vi "LoadIRF.vi"(8 "error in (no error)":errorcluster, 11 "file path":path=path "C:/Users/MarcuAdmin/Documents/GitHub/NetDeconForLV/Testing/irf files/Channel1.tdms") -> (0 "error out":errorcluster, 3 "APD":T1)   [LabVIEW 2020]
uses:
  APD.ctl
  <vilib>/Utility/TDMS File Viewer/NI_TDMS File Viewer.lvlib
panel:
  out "WFLength":i32
  out "Waveform Graph":dbl[][](graph)
  out "XY Graph":cluster{dbl[], dbl[]}(graph)
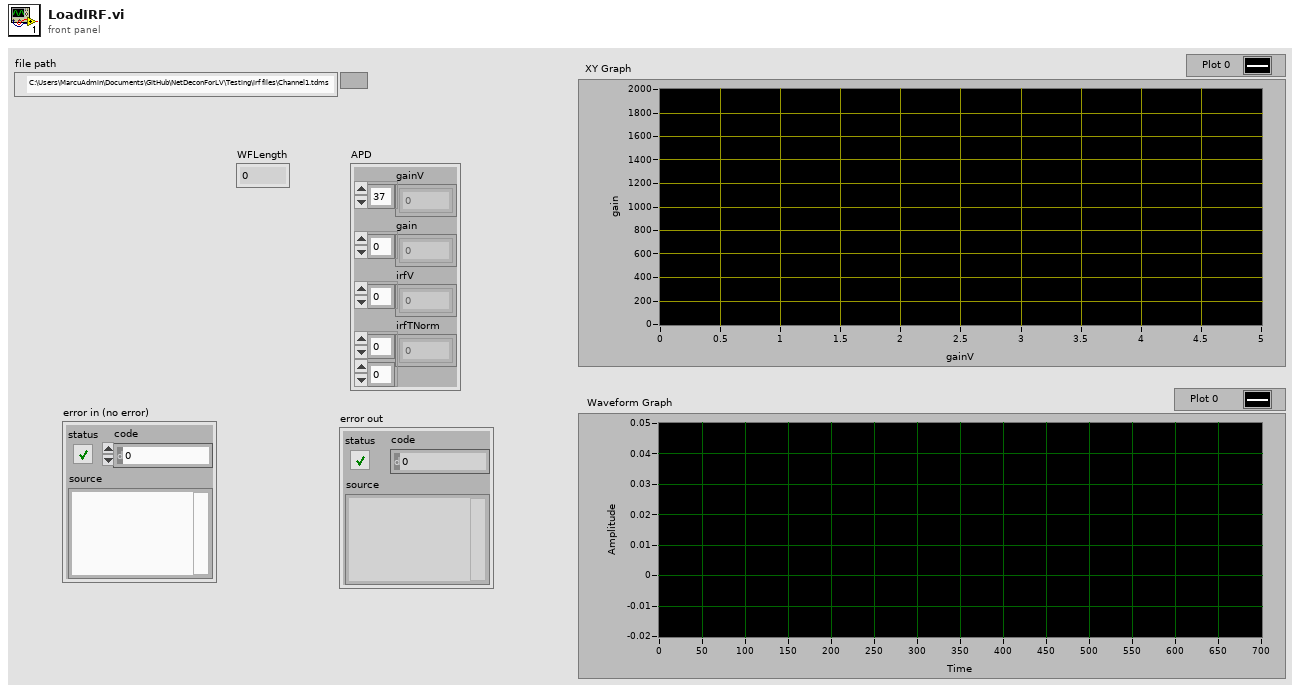
[diagram p1: front panel]
types:
  T1 = typedef "APD.ctl" = cluster{"gainV":dbl[], "gain":dbl[], "irfV":dbl[], "irfTNorm":dbl[][]}
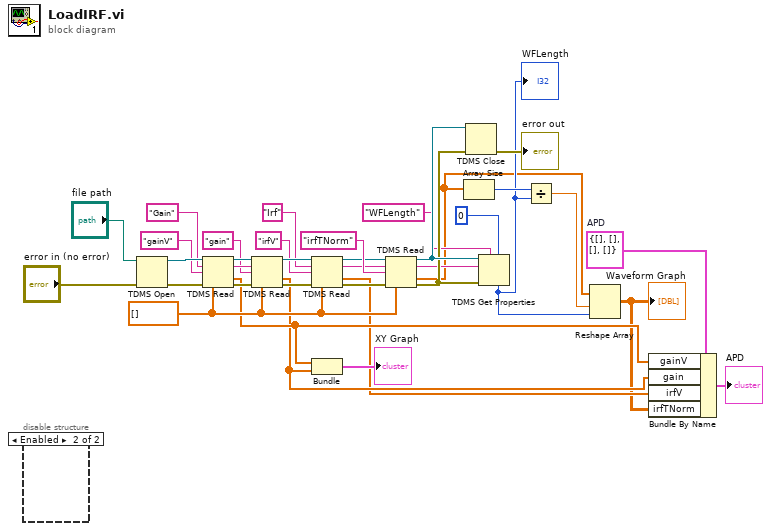
[diagram p0: block diagram]
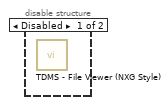
[diagram p2: hidden frame]
diagram:
  w7 = T1 {"gainV"=[], "gain"=[], "irfV"=[], "irfTNorm"=[]}  # APD
  w19 = dbl[] []
  n1 = disable-structure shown="Enabled" {
    frame Disabled {
      n2 = call <vilib>:"TDMS - File Viewer (NXG Style).vi"() -> ()  [unwired: 10 in, 2 out]
    }
    frame Enabled {
    }
  }
  n3 = TDMS Open(8:"error in (no error)", 11:"file path") -> (0:w33:errorcluster, 3:w36:refnum<k34>)  [unwired: 5 in]
  n4 = TDMS Read(0:w36, 5:"Gain" ("group name in"), 7:"gainV" ("channel name(s) in"), 11:w33, 12:w19) -> (4:w29:refnum<k34>, 6:w28:string, 10:w6:dbl[], 15:w27:errorcluster)  [unwired: 3 in, 2 out]
  n5 = TDMS Read(0:w29, 5:w28, 7:"gain" ("channel name(s) in"), 11:w27, 12:w19) -> (4:w25:refnum<k34>, 10:w5:dbl[], 15:w24:errorcluster)  [unwired: 3 in, 3 out]
  n6 = TDMS Read(0:w25, 5:"Irf" ("group name in"), 7:"irfV" ("channel name(s) in"), 11:w24, 12:w19) -> (4:w17:refnum<k34>, 6:w18:string, 10:w4:dbl[], 15:w16:errorcluster)  [unwired: 3 in, 2 out]
  n7 = Bundle(w6, w5) -> (→"XY Graph":cluster{dbl[], dbl[]})  [unwired: 1 in]
  n8 = TDMS Read(0:w17, 5:w18, 7:"irfTNorm" ("channel name(s) in"), 11:w16, 12:w19) -> (4:w15:refnum<k34>, 6:w13:string, 10:w3:dbl[], 15:w14:errorcluster)  [unwired: 3 in, 2 out]
  n9 = Array Size(array=w3) -> (size(s)=w10:i32)
  n10 = TDMS Close(8:w14, 11:w15) -> (0:→"error out":errorcluster)  [unwired: 1 out]
  n11 = TDMS Get Properties(5:0, 7:"WFLength" ("property name"), 8:w14, 10:w13, 11:w15) -> (4:w9:i32)  [unwired: 1 in, 5 out]
  "WFLength" <- w9
  n12 = Divide(x=w10, y=w9) -> (x/y=w8:dbl)
  n13 = Reshape Array(w3, w8, w9) -> (w2:dbl[][])
  "Waveform Graph" <- w2
  n14 = Bundle By Name(cluster=w7, "gainV"=w6, "gain"=w5, "irfV"=w4, "irfTNorm"=w2) -> (→"APD":T1)
